vi "NI Detection_One.vi"() -> (0 "NI 2":tag, 1 "NI 1":tag, 2 "Ok/Cancel":enum16{"Ok", "Cancel"}(ring))   [LabVIEW 2017]
uses:
  <resource>/objmgr/daqmx.rc
panel:
  in  "NI":tag
  in  "Cancel Button":bool
  in  "OK Button":bool
  # "PLease Choose Correct NI Serial Number"
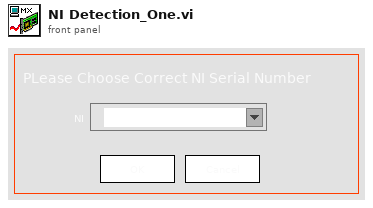
[diagram p1: front panel]
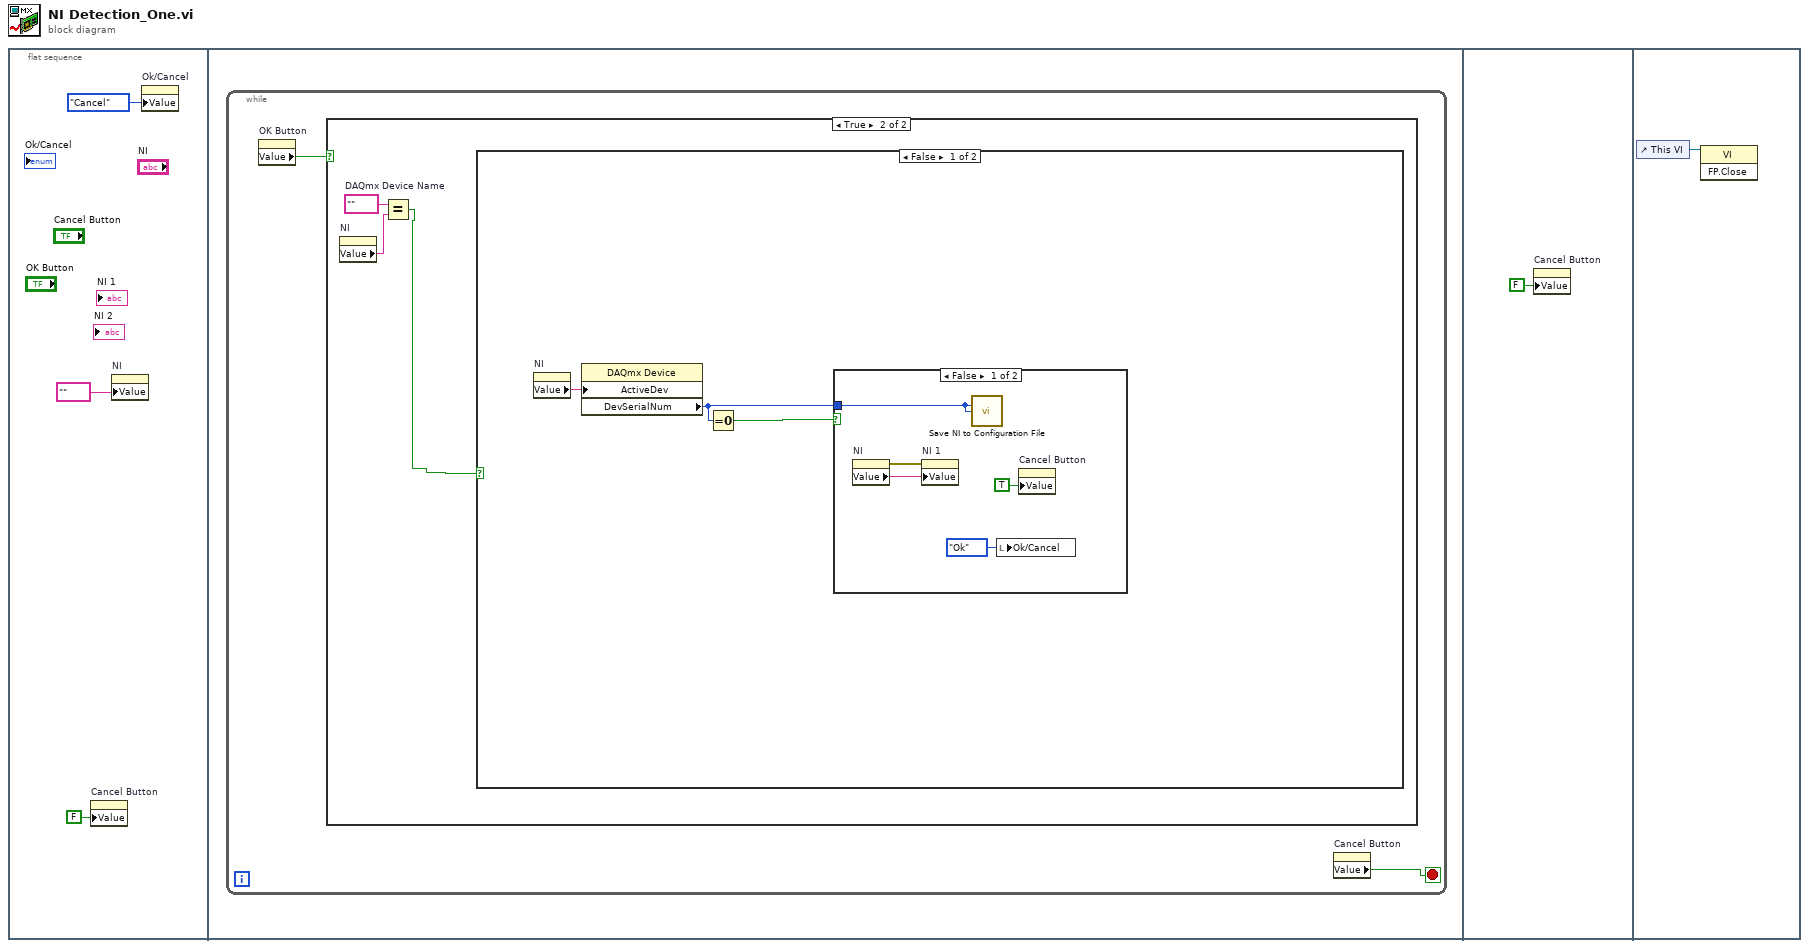
[diagram p0: block diagram]
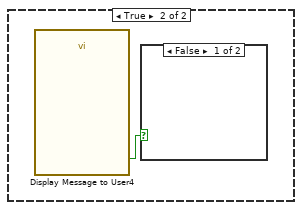
[diagram p3: hidden frame]
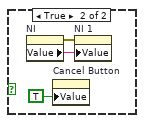
[diagram p4: hidden frame]
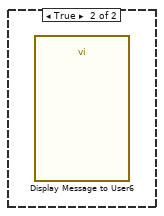
[diagram p5: hidden frame]
diagram:
  n1 = flat-sequence {
    frame #0 {
      n2 = property on="Cancel Button" class="Bool (strict)"("Value"=FALSE ("Cancel Button")) -> ()  [unwired: 2 in, 2 out]
      n3 = property on="NI" class="DAQmxName"("Value"=tag "" ("NI 2")) -> ()  [unwired: 2 in, 2 out]
      n4 = property on="Ok/Cancel" class="Enum (strict)"("Value"=enum16{"Ok", "Cancel"}."Cancel" ("Ok/Cancel")) -> ()  [unwired: 2 in, 2 out]
    }
    frame #1 {
      n5 = while {
        stop <- w4 stop-if-true
        n6 = property on="OK Button" class="Bool (strict)"() -> ("Value"=w5:bool)  [unwired: 2 in, 2 out]
        n7 = case shown="True" w5 {
          frame False {
          }
          frame True {
            w8 = tag ""  # DAQmx Device Name
            n8 = property on="NI" class="DAQmxName"() -> ("Value"=w7:string)  [unwired: 2 in, 2 out]
            n9 = Equal?(x=w8, y=w7) -> (x = y?=w6:bool)
            n10 = case shown="False" w6 {
              frame False {
                n11 = property on="NI" class="DAQmxName"() -> ("Value"=w11:string)  [unwired: 2 in, 2 out]
                n12 = property class="DAQmx Device"("ActiveDev"=w11) -> ("DevSerialNum"=w9:u32)  [unwired: 2 in, 2 out]
                n13 = Equal To 0?(x=w9) -> (x = 0?=w10:bool)
                n14 = case shown="False" w10 {
                  tunnel: w9 -> [w12 _]
                  frame False {
                    n15 = property on="NI" class="DAQmxName"() -> (error out=w16:errorcluster, "Value"=w15:string)  [unwired: 2 in, 1 out]
                    n16 = property on="NI 1" class="DAQmxName"(error in=w16, "Value"=w15) -> ()  [unwired: 1 in, 2 out]
                    n17 = call "Save NI to Configuration File.vi"("NI1"=w12, "NI2"=w12) -> ()  [unwired: 14 in]
                    n18 = local write "Ok/Cancel"(enum16{"Ok", "Cancel"}."Ok" ("Ok/Cancel")) -> ()
                    n19 = property on="Cancel Button" class="Bool (strict)"("Value"=TRUE ("Cancel Button")) -> ()  [unwired: 2 in, 2 out]
                  }
                  frame True {
                    n20 = call "Display Message to User4"() -> ("OK"=w17:bool)  [unwired: 10 in, 1 out]
                    n21 = case shown="False" w17 {
                      frame False {
                      }
                      frame True {
                        n22 = property on="NI" class="DAQmxName"() -> (error out=w20:errorcluster, "Value"=w19:string)  [unwired: 2 in, 1 out]
                        n23 = property on="Cancel Button" class="Bool (strict)"("Value"=TRUE ("Cancel Button")) -> ()  [unwired: 2 in, 2 out]
                        n24 = property on="NI 1" class="DAQmxName"(error in=w20, "Value"=w19) -> ()  [unwired: 1 in, 2 out]
                      }
                    }
                  }
                }
              }
              frame True {
                n25 = call "Display Message to User6"() -> ()  [unwired: 10 in, 2 out]
              }
            }
          }
        }
        n26 = property on="Cancel Button" class="Bool (strict)"() -> ("Value"=w4:bool)  [unwired: 2 in, 2 out]
      }
    }
    frame #2 {
      n27 = property on="Cancel Button" class="Bool (strict)"("Value"=FALSE ("Cancel Button")) -> ()  [unwired: 2 in, 2 out]
    }
    frame #3 {
      n28 = control-ref of="This VI"() -> (w22:refnum<vi>)
      n29 = invoke class="VI" method="FP.Close"(reference=w22) -> ()  [unwired: 2 in, 3 out]
    }
  }
